vi "缺陷评定辅助信息输入子VI.vi"() -> (3 "评定辅助信息":T1)   [LabVIEW 2018]
panel:
  in  "确定按钮":bool
  in  "结果评定辅助信息":T1={"分层类缺陷验收要求（Z值）"=13.0, "弥散类缺陷验收要求（%）"=10.0, "弥散类缺陷评定矩形面积"=20.0, "认定缺陷阈值"=10.0} {"认定缺陷阈值" format="%#_g%%"; "弥散类缺陷评定矩形面积" format="%#_6f"; "弥散类缺陷验收要求（%）" format="%#_g%%"}
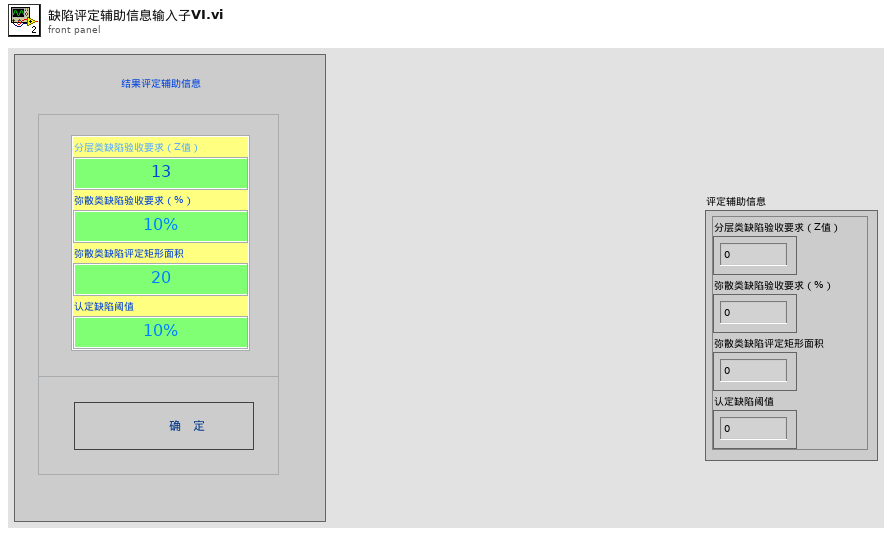
[diagram p1: front panel]
types:
  T1 = cluster{"分层类缺陷验收要求（Z值）":dbl, "弥散类缺陷验收要求（%）":dbl, "弥散类缺陷评定矩形面积":dbl, "认定缺陷阈值":dbl}
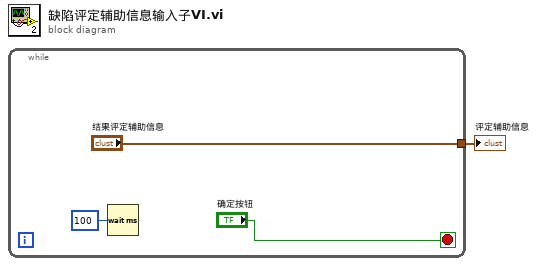
[diagram p0: block diagram]
diagram:
  n1 = while {
    tunnel: ["结果评定辅助信息"] -> w1
    stop <- "确定按钮" stop-if-true
    n2 = Wait (ms)(milliseconds to wait=u32 100 ("等待时间（毫秒）")) -> ()  [unwired: 1 out]
  }
  "评定辅助信息" <- w1
